vi "传输数据.vi"(4 "纵轴数组":i32[](array[numeric]), 6 "横纵数组":i32[](array[numeric]), 7 "输出簇":cluster{"是否手动取点":bool, "手动取点x":i32, "手动取点y":i32}, 8 "error in (no error)":errorcluster, 9 "阈值等级":i32=4, 10 "配置缓存":T3, 11 "Image Src":T1) -> (0 "error out":errorcluster, 1 "灰度图像":T1, 3 "已采集数据":T2)   [LabVIEW 2015]
uses:
  <vilib>/vision/Image Controls.llb/IMAQ Image.ctl
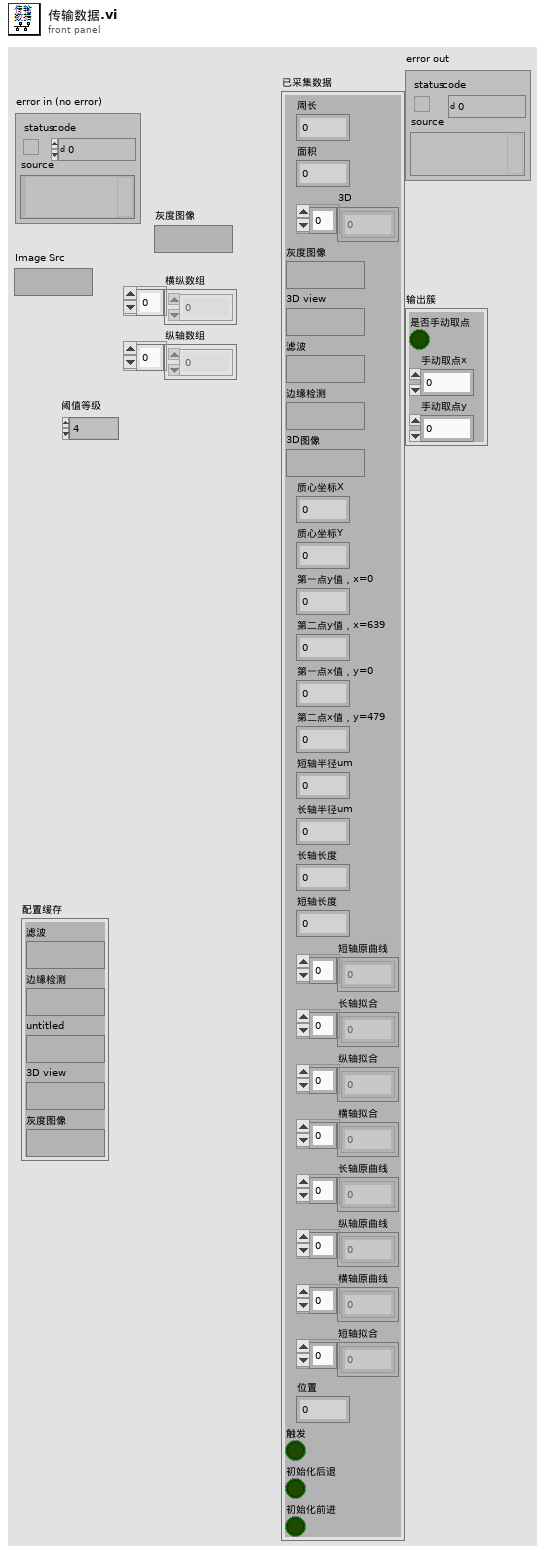
[diagram p1: front panel]
types:
  T1 = typedef "IMAQ Image.ctl" = refnum<image>
  T2 = cluster{"周长":dbl, "面积":dbl, "3D":u8[], "灰度图像":T1, "3D view":T1, "滤波":T1, "边缘检测":T1, "3D图像":T1, "质心坐标X":sgl, "质心坐标Y":sgl, "第一点y值，x=0":dbl, "第二点y值，x=639":dbl, "第一点x值，y=0":dbl, "第二点x值，y=479":dbl, "短轴半径um":dbl, "长轴半径um":dbl, "长轴长度":dbl, "短轴长度":dbl, "短轴原曲线":dbl[], "长轴拟合":dbl[], "纵轴拟合":dbl[], "横轴拟合":dbl[], "长轴原曲线":dbl[], "纵轴原曲线":dbl[], "横轴原曲线":dbl[], "短轴拟合":dbl[], "位置":dbl, "触发":bool, "初始化后退":bool, "初始化前进":bool}
  T3 = cluster{"滤波":T1, "边缘检测":T1, "untitled":T1, "3D view":T1, "灰度图像":T1}
  T4 = cluster{"Center":cluster{"X":sgl, "Y":sgl}, "Major Axis":cluster{"Point 1":cluster{"X":sgl, "Y":sgl}, "Point 2":cluster{"X":sgl, "Y":sgl}}, "Minor Axis":cluster{"Point 1":cluster{"X":sgl, "Y":sgl}, "Point 2":cluster{"X":sgl, "Y":sgl}}}
  T5 = cluster{"Point 1":cluster{"X":sgl, "Y":sgl}, "Point 2":cluster{"X":sgl, "Y":sgl}}
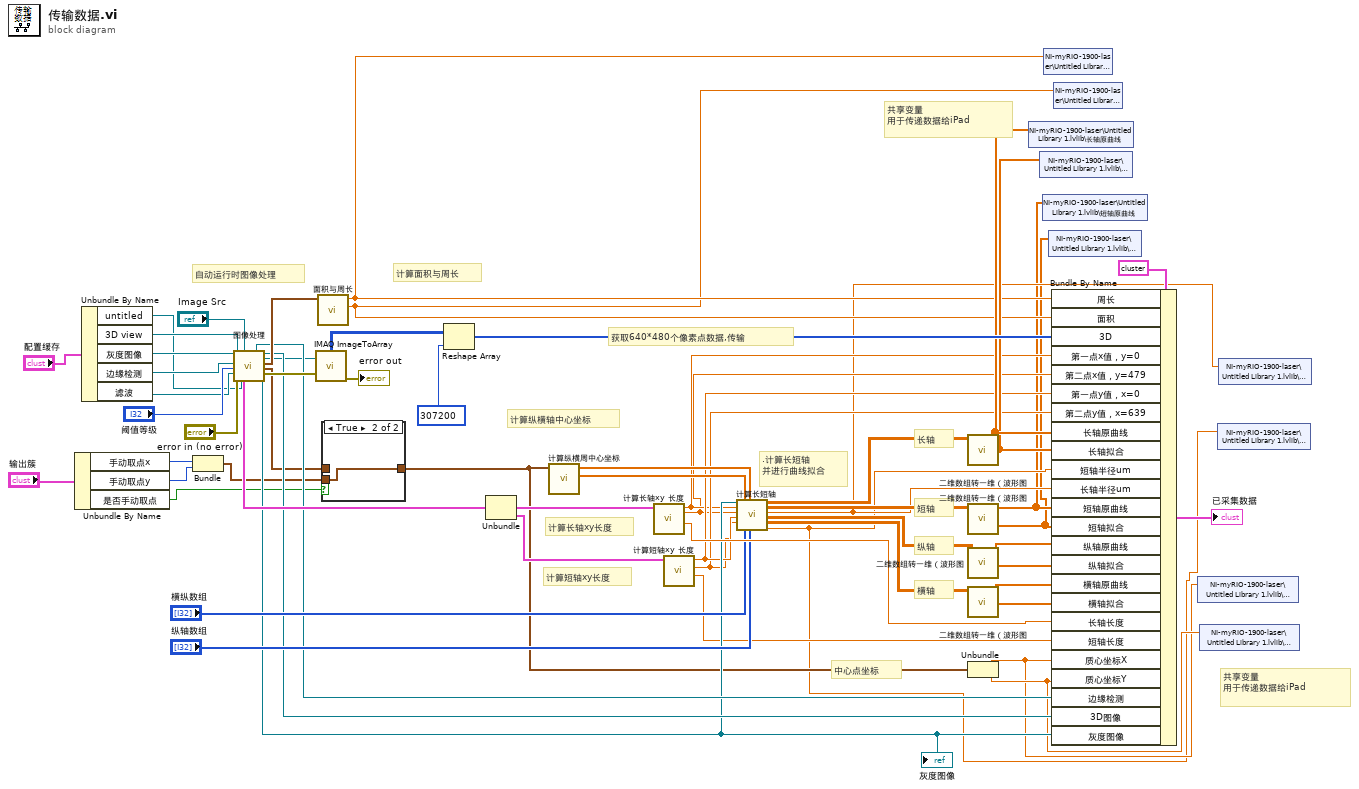
[diagram p0: block diagram]
diagram:
  # "共享变量\n用于传递数据给iPad"
  # "共享变量\n用于传递数据给iPad"
  # "自动运行时图像处理"
  # "中心点坐标"
  # "短轴"
  # "长轴"
  # "横轴"
  # "纵轴"
  # ".计算长短轴\n并进行曲线拟合"
  # "计算短轴xy长度"
  # "计算长轴xy长度"
  # "计算纵横轴中心坐标"
  # "计算面积与周长"
  # "获取640*480个像素点数据,传输"
  n1 = Unbundle By Name("输出簇") -> ("手动取点x"=w17:i32, "手动取点y"=w16:i32, "是否手动取点"=w18:bool)
  n2 = Unbundle By Name("配置缓存") -> ("untitled"=w3:T1, "3D view"=w55:T1, "灰度图像"=w54:T1, "边缘检测"=w53:T1, "滤波"=w52:T1)
  n3 = Bundle("手动取点x"=w17, "手动取点y"=w16) -> (w15:cluster{"手动取点x":i32, "手动取点y":i32})  [unwired: 1 in]
  n4 = call "图像处理.vi"("imaq creat"=w54, "Image Src"="Image Src", "边缘检测"=w53, "Number of Classes"="阈值等级", "滤波"=w52, "error in (no error)"="error in (no error)", "3D view"=w55, "United"=w3) -> ("overlay"=w30:T1, "Ellipse"=w40:T4, "3D"=w29:T1, "灰度图像"=w28:T1, "Measurements"=w57:cluster{"Area":dbl, "Perimeter":dbl}, "Centroid"=w20:cluster{"X Centroid":sgl, "Y Centroid":sgl}, "error out"=w56:errorcluster)  [unwired: 5 in]
  "灰度图像" <- w28
  n5 = call "IMAQ ImageToArray"("error in (no error)"=w56, "Image"=w28) -> ("error out"=→"error out":errorcluster, "Image Pixels (U8)"=w50:u8[][])  [unwired: 2 in, 3 out]
  n6 = call "面积与周长.vi"("测量结果"=w57) -> ("周长"=w22:dbl, "面积"=w23:dbl)  [unwired: 9 in]
  n7 = case shown="True" w18 {
    tunnel: w20 -> [w59 _]
    tunnel: [w59 w60] -> w19
    tunnel: w15 -> [_ w60]
    frame False {
    }
    frame True {
    }
  }
  n8 = Reshape Array(w50, 307200 ("dimension size")) -> (w49:u8[])
  n9 = Unbundle(w40) -> ("Major Axis"=w47:T5, "Minor Axis"=w48:T5)  [unwired: 1 out]
  n10 = call "计算纵横周中心坐标.vi"("Center"=w19) -> ("所在直线 纵"=w46:sgl[], "所在直线 横"=w45:sgl[])  [unwired: 9 in]
  n11 = call "计算长轴xy 长度.vi"("Major Axis"=w47) -> ("长轴长度"=w39:dbl, "第二点x值，y=479"=w9:dbl, "第一点x值，y=0"=w10:dbl)  [unwired: 8 in]
  n12 = call "计算短轴xy 长度.vi"("Minor Axis"=w48) -> ("短轴长度"=w12:dbl, "第二点y值，x=639"=w11:dbl, "第一点y值，x=0"=w13:dbl)  [unwired: 8 in]
  n13 = call "计算长短轴.vi"("灰度图像"=w28, "第一点x值，y=0"=w10, "第二点x值，y=479"=w9, "第一点y值，x=0"=w13, "第二点y值，x=639"=w11, "所在直线 纵"=w46, "横纵数组"="横纵数组", "所在直线 横"=w45, "纵轴数组"="纵轴数组") -> ("长轴"=w43:dbl[][], "短轴"=w42:dbl[][], "长轴半径um"=w6:dbl, "纵轴"=w44:dbl[][], "横轴"=w41:dbl[][], "短轴半径um"=w5:dbl)  [unwired: 5 in]
  n14 = call "二维数组转一维（波形图.vi"("二维数组"=w43) -> ("第二列"=w31:dbl[], "第一列"=w32:dbl[])  [unwired: 9 in]
  n15 = call "二维数组转一维（波形图.vi"("二维数组"=w42) -> ("第二列"=w1:dbl[], "第一列"=w2:dbl[])  [unwired: 9 in]
  n16 = call "二维数组转一维（波形图.vi"("二维数组"=w44) -> ("第二列"=w26:dbl[], "第一列"=w27:dbl[])  [unwired: 9 in]
  n17 = call "二维数组转一维（波形图.vi"("二维数组"=w41) -> ("第二列"=w24:dbl[], "第一列"=w25:dbl[])  [unwired: 9 in]
  n18 = Unbundle(w19) -> ("X Centroid"=w7:sgl, "Y Centroid"=w8:sgl)
  n19 = shared-variable "NI-myRIO-1900-laser\\Untitled Library 1.lvlib\\长轴原曲线"(w32) -> ()  [unwired: 1 in, 1 out]
  n20 = shared-variable "NI-myRIO-1900-laser\\Untitled Library 1.lvlib\\长轴拟合"(w31) -> ()  [unwired: 1 in, 1 out]
  n21 = shared-variable "NI-myRIO-1900-laser\\Untitled Library 1.lvlib\\短轴原曲线"(w2) -> ()  [unwired: 1 in, 1 out]
  n22 = shared-variable "NI-myRIO-1900-laser\\Untitled Library 1.lvlib\\周长"(w23) -> ()  [unwired: 1 in, 1 out]
  n23 = shared-variable "NI-myRIO-1900-laser\\Untitled Library 1.lvlib\\短轴拟合"(w1) -> ()  [unwired: 1 in, 1 out]
  n24 = Bundle By Name(cluster=T2 {"周长"=0.0, "面积"=0.0, "3D"=[], "灰度图像"=refnum, "3D view"=refnum, "滤波"=refnum, "边缘检测"=refnum, "3D图像"=refnum, "质心坐标X"=0.0, "质心坐标Y"=0.0, "第一点y值，x=0"=0.0, "第二点y值，x=639"=0.0, "第一点x值，y=0"=0.0, "第二点x值，y=479"=0.0, "短轴半径um"=0.0, "长轴半径um"=0.0, "长轴长度"=0.0, "短轴长度"=0.0, "短轴原曲线"=[], "长轴拟合"=[], "纵轴拟合"=[], "横轴拟合"=[], "长轴原曲线"=[], "纵轴原曲线"=[], "横轴原曲线"=[], "短轴拟合"=[], "位置"=0.0, "触发"=TRUE, "初始化后退"=TRUE, "初始化前进"=TRUE}, "周长"=w23, "面积"=w22, "3D"=w49, "第一点x值，y=0"=w10, "第二点x值，y=479"=w9, "第一点y值，x=0"=w13, "第二点y值，x=639"=w11, "长轴原曲线"=w32, "长轴拟合"=w31, "短轴半径um"=w5, "长轴半径um"=w6, "短轴原曲线"=w2, "短轴拟合"=w1, "纵轴原曲线"=w27, "纵轴拟合"=w26, "横轴原曲线"=w25, "横轴拟合"=w24, "长轴长度"=w39, "短轴长度"=w12, "质心坐标X"=w7, "质心坐标Y"=w8, "边缘检测"=w30, "3D图像"=w29, "灰度图像"=w28) -> (→"已采集数据":T2)
  n25 = shared-variable "NI-myRIO-1900-laser\\Untitled Library 1.lvlib\\面积"(w22) -> ()  [unwired: 1 in, 1 out]
  n26 = shared-variable "NI-myRIO-1900-laser\\Untitled Library 1.lvlib\\质心坐标X"(w7) -> ()  [unwired: 1 in, 1 out]
  n27 = shared-variable "NI-myRIO-1900-laser\\Untitled Library 1.lvlib\\质心坐标Y"(w8) -> ()  [unwired: 1 in, 1 out]
  n28 = shared-variable "NI-myRIO-1900-laser\\Untitled Library 1.lvlib\\短轴半径"(w5) -> ()  [unwired: 1 in, 1 out]
  n29 = shared-variable "NI-myRIO-1900-laser\\Untitled Library 1.lvlib\\长轴半径"(w6) -> ()  [unwired: 1 in, 1 out]
